vi "Parse and Prep Waypoint config file.vi"(8 "error in (no error)":errorcluster, 11 "Waypoint Dictionary ConfigFile":path=path "C:/Projects/BRS_Dev/BRS Information/Waypoint Dictionary Configuration File.xml") -> (0 "error out":errorcluster, 1 "WyPtFullNode[]":T4[](array[typedef]), 2 "CmdNumber[]":string[](array[string]), 3 "Handshake[]":T2[](array[typedef]), 4 "WyPtDictNode[]":T1[](array[typedef]))   [LabVIEW 2020, in "WyPtDict.lvlib"]
uses:
  WyPtDict.lvlib
  WyPtFullNode--cluster.ctl
  RoboWaypointDict Node--cluster.ctl
  BRS_Dev/Source Code/Robo Driver/Controls/MC and Robo Handshake.ctl
  StockerExpansionModuleID--enum.ctl
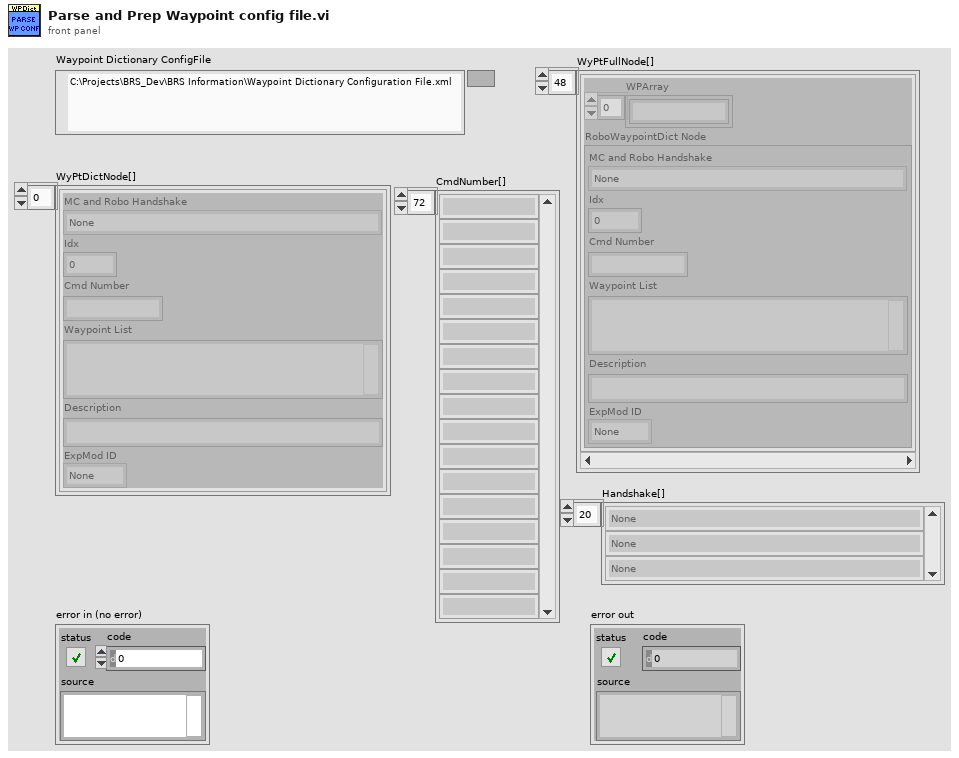
[diagram p1: front panel]
types:
  T1 = typedef "WyPtDict.lvlib/RoboWaypointDict Node--cluster.ctl" = cluster{"MC and Robo Handshake":T2, "Idx":i32, "Cmd Number":string, "Waypoint List":string, "Description":string, "ExpMod ID":T3}
  T2 = typedef "MC and Robo Handshake.ctl" = enum16{"None", "Move and Pick Nikon Ret LP(1100)", "Nikon Barcode1 Scanning Started(1101)", "Nikon Barcode1 Scan Abort(1102)", "Nikon Barcode1 Scan Success Proc to Barcode 2 Pos(1103)", "Nikon Barcode 2 Scanning Started(1104)", "Nikon Barcode 2 Scan Abort(1105) ", "Nikon Barcode 2 Success(1106)", "Move and Pick POZZ Ret LP(1300)", "POZZ Barcode Scan Started(1301)", "POZZ Barcode Not Found(1302)", "POZZ Barcode Scan Succ(1303)", "POZZ Mov to Side 2 Bar 2(1310)", "POZZ Mov to Side 4 Bar 1(1311)", "POZZ Mov to Side 4 Bar 2(1312)", "POZZ Mov to Side 1 Bar 1(1313)", "POZZ Mov to Side 1 Bar 2(1314)", "POZZ Mov to Side 3 Bar 1(1315)", "POZZ Mov to Side 3 Bar 2(1316)", "POZZ Mov to Edge 3 Nik 2(1317)", "POZZ Mov to Edge 4 ASML(1318)", "POZZ Mov to Edge 4 Nik 1(1319)", "Check BC 180 Position(1320)", "Move to ASML LP and Pick Ret(2000)", "ASML1 Barcode Scan Started(2001)", "ASML1 Barcode Not Found(2002)", "ASML1 Barcode Scan Succ(2003)", "Start Load Seq for Nikon LP(3000)", "Start Load Seq for POZZ LP(3200)", "Start Load Seq for ASML LP(3400)", "Start Align End Grip Place Func(4000)", "Start Align End grip Pick Func(4001)", "Start Align Center Grip Place Func(4002)", "Start Align Center grip Pick Func(4003)", "Start Move from home to Cleaner(5000)", "Start Move to Final Cleaner Loc(5001)", "Start Move to Initial Cleaner Loc(5002)", "Start Move from home to PDS for Inspect(6000) ", "PDS Inspect Finished(6001)", "PDS EMO Recovery(6002)", "Store in Stocker(7001)", "Store in Exp1 Stocker(7402)", "Retrive from Center Stocker(8001)", "Retrive Mov to Nikon BC1 Scan Pos(8002)", "Retrive Nikon BC1not found(8003)", "Retrive Nikon BC1 Scan Succ(8004)", "Retrive Nikon BC2 not found(8005)", "Retrive Nikon BC2 scan Succ(8006)", "Retrive Mov to Edge 1 ASML(8202) ", "Retrive Mov to Edge 1 Nikon 1(8203)", "Retrive Mov to Edge 1 Nikon 2(8204)", "Retrive Mov to Edge 2 ASML(8205)", "Retrive Mov to Edge 2 Nikon 1(8206)", "Retrive Mov to Edge 2 Nikon 2(8207)", "Retrive Mov to Edge 3 ASML (8208)", "Retrive Mov to Edge 3 Nikon 1(8209)", "Retrive Mov to Edge 3 Nikon 2(8210)", "Retrive Mov to Edge 4 ASML (8211)", "Retrive Mov to Edge 4 Nikon 1 (8212)", "Retrive Mov to Edge 4 Nikon 2 (8213)", "Retrive BC Scan Abort (8214)", "Retrive BC Scan Successful (8215)", "Retrive Mov to ASML BC scan Pos (8402) ", "Retrive ASML BC not found(8403)", "Retrive ASML BC Scan Succ(8404)", "Exp1 Retrive Seq (8602)", "Cen Stocker move from home to Transit Nest(9000)", "Cen Stocker move from Transit Nest to home(9200)", "Exp1 Stocker move from home to Transit Nest(9400)", "Exp1 Stocker move from Transit Nest to home(9600)", "Move to R1 Home (1000)", "Move to R2 Home (1111)", "Store Left Stocker (7401)", "Retrieve Left Stocker (8601)", "EMO Recovery Center (1002)", "EMO Recovery Exp1 (1003)", "Center Robo Status (8888)", "Exp1 Robo Status (8889)", "Exp2 move from home to Transit Nest (9500)", "Exp2 move from Transit Nest to home (9700)", "Move to R3 Home (2222)", "Store Exp2 (7501)", "Retrieve Exp2 (8701)", "Exp2 Robo Status (8887)", "EMO Recovery Exp2 (1004)", "Move to ASML LP and Pick Ret NikFmt(2004)", "Move to Diagonal BC Scan Loc (8010)", "Start Move from Cleaner loc to home(5003)"}
  T3 = typedef "WyPtDict.lvlib/StockerExpansionModuleID--enum.ctl" = enum16{"None", "Main", "Exp1", "Exp2", "Exp3", "Exp4", "Exp5"}
  T4 = typedef "WyPtDict.lvlib/WyPtFullNode--cluster.ctl" = cluster{"WPArray":string[], "RoboWaypointDict Node":T1}
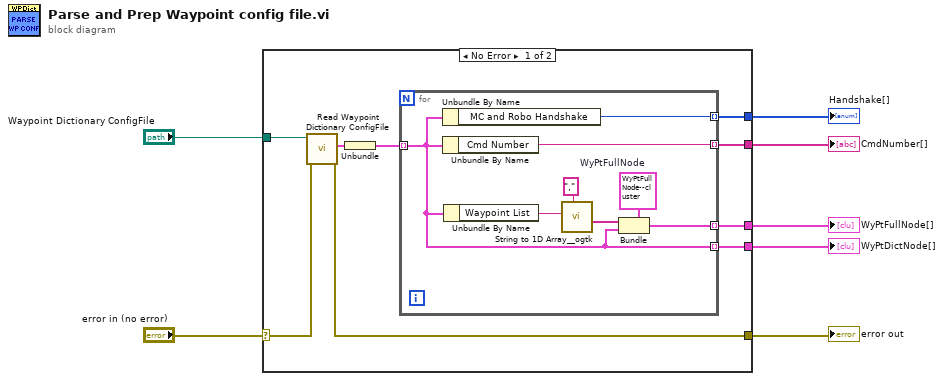
[diagram p0: block diagram]
diagram:
  n1 = case shown="No Error" "error in (no error)" {
    selector: "error in (no error)" -> [w9 w25]
    tunnel: "Waypoint Dictionary ConfigFile" -> [w16 _]
    tunnel: [w13 _] -> w6
    tunnel: [w12 _] -> w5
    tunnel: [w11 _] -> w4
    tunnel: [w10 w25] -> w3
    tunnel: [w8 _] -> w1
    frame No Error {
      n2 = call "Read Waypoint Dictionary ConfigFile.vi"("error in (no error)"=w9, "Waypoint Dictionary ConfigFile"=w16) -> ("error out"=w10:errorcluster, "WaypointDictionary"=w15:cluster{"WyPtDictNode":T1[]})  [unwired: 7 in, 1 out]
      n3 = Unbundle(w15) -> ("WyPtDictNode"=w14:T1[])
      n4 = for {
        tunnel: w14 -> [w17] mode=indexing
        tunnel: [w24] -> w11 mode=indexing
        tunnel: [w23] -> w12 mode=indexing
        tunnel: [w18] -> w13 mode=indexing
        tunnel: [w17] -> w8 mode=indexing
        w19 = T4 {"WPArray"=[], "RoboWaypointDict Node"={"MC and Robo Handshake"=enum."None", "Idx"=0, "Cmd Number"="", "Waypoint List"="", "Description"="", "ExpMod ID"=enum."None"}}  # WyPtFullNode
        n5 = Unbundle By Name(w17) -> ("MC and Robo Handshake"=w24:T2)
        n6 = Unbundle By Name(w17) -> ("Cmd Number"=w23:string)
        n7 = Unbundle By Name(w17) -> ("Waypoint List"=w22:string)
        n8 = call <userlib>:"String to 1D Array__ogtk.vi"("delimiter (Tab)"=",", "string"=w22) -> ("Array of Strings"=w20:string[])  [unwired: 9 in]
        n9 = Bundle(cluster=w19, "WPArray"=w20, "RoboWaypointDict Node"=w17) -> (w18:T4)
      }
    }
    frame Error {
    }
  }
  "WyPtFullNode[]" <- w6
  "CmdNumber[]" <- w5
  "Handshake[]" <- w4
  "error out" <- w3
  "WyPtDictNode[]" <- w1
